vi "Wrapper_AgentGpgCryption.vi"(2 "data string":string, 5 "error in (no error)":errorcluster, 7 "receiver ID":string, 8 "task":enum16{"encrypt", "decrypt", "sign", "verify"}(ring), 9 "HGF_Agent":refnum<class "MoAgSy_AgentBase.lvclass">) -> (16 "String out":string, 17 "success":bool, 19 "error out":errorcluster)   [LabVIEW 2009, in "MoAgSy.lvlib"]
doc: "Wrapper VI for Agent's GPG Cryption functions.\nOnly executes if MoAgSy_StateMachine is part of the call chain.\nNeeded, because statechart is incompatible with friends.\n\nF.Berck@gsi.de\nGSI Darmstadt 2009"
uses:
  MoAgSy.lvlib
  MoAgSy_AgentBase/MoAgSy_AgentBase.lvclass
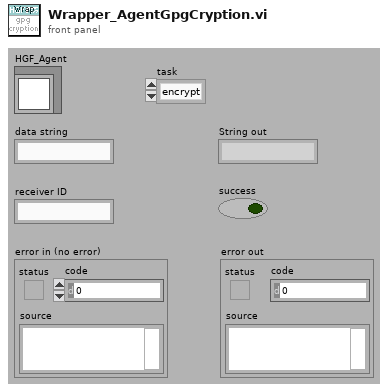
[diagram p1: front panel]
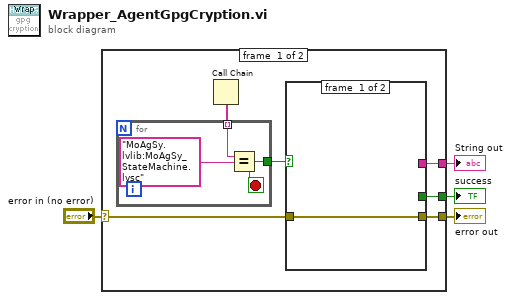
[diagram p0: block diagram]
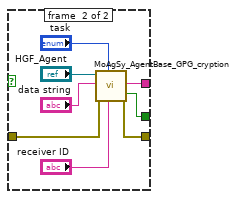
[diagram p2: hidden frame]
diagram:
  n1 = case shown="No Error" "error in (no error)" {
    selector: "error in (no error)" -> [w8 w23]
    tunnel: [w10 w23] -> w4
    tunnel: [w6 _] -> w2
    tunnel: [w5 _] -> w1
    frame #0 {
      n2 = Call Chain() -> (call chain=w9:string[])
      n3 = for {
        tunnel: w9 -> [w12] mode=indexing
        tunnel: [w11] -> w7
        stop <- w11 stop-if-true
        n4 = Equal?(x=w12, y="MoAgSy.lvlib:MoAgSy_StateMachine.lvsc") -> (x = y?=w11:bool)
      }
      n5 = case shown="True" w7 {
        tunnel: [w14 w22] -> w10
        tunnel: [_ w21] -> w5
        tunnel: [_ w20] -> w6
        tunnel: w8 -> [w14 w15]
        frame #0 {
        }
        frame #1 {
          n6 = call "MoAgSy_AgentBase_GPG_cryption.vi"("HGF_Agent in"="HGF_Agent", "string in"="data string", "error in (no error)"=w15, "task"="task", "receiver"="receiver ID") -> ("String out"=w21:string, "success"=w20:bool, "error out"=w22:errorcluster)  [unwired: 11 in, 1 out]
        }
      }
    }
    frame #1 {
    }
  }
  "error out" <- w4
  "String out" <- w1
  "success" <- w2
